vi "ManipWait.vi"(2 "Time Since Latch":u32, 3 "Instruction String":string) -> (0 "Error Out":errorcluster, 1 "Advance Trigger":bool)   [LabVIEW 2019]
uses:
  SafeParser_Integer.vi
  SafeParser_Float.vi
  SafeParser_String.vi
  dsdata.vi
  autoninfo.vi
  outputs.vi
  sensors.vi
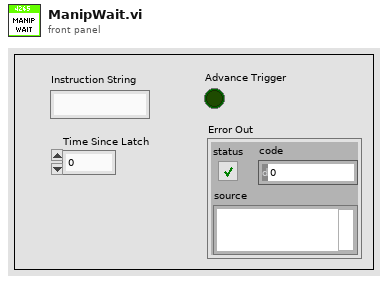
[diagram p1: front panel]
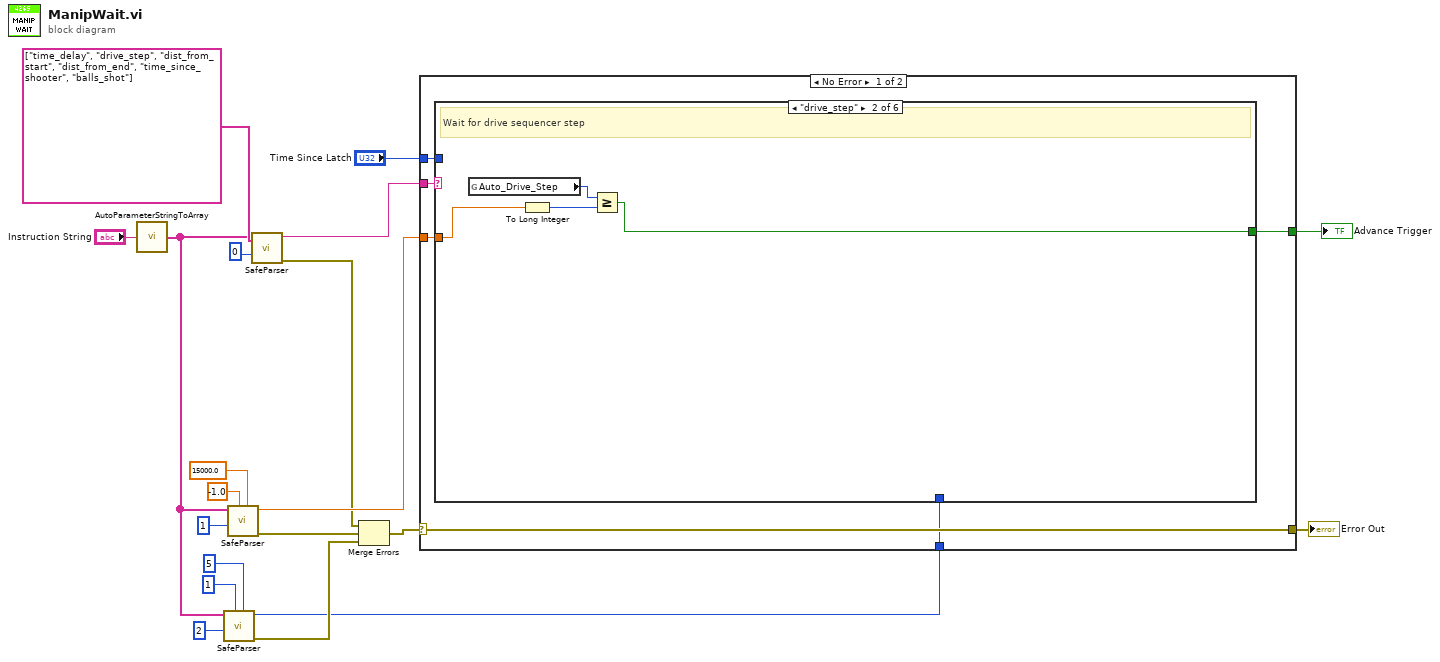
[diagram p0: block diagram]
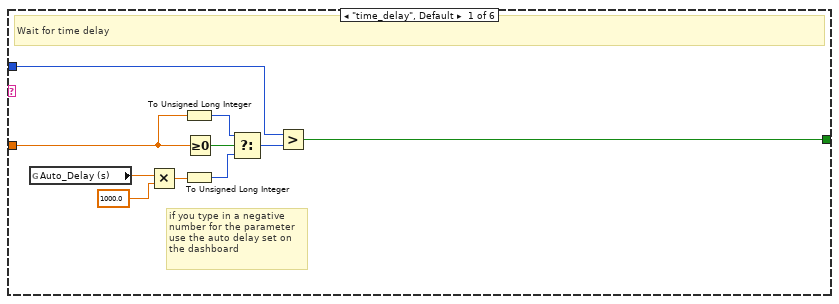
[diagram p2: hidden frame]
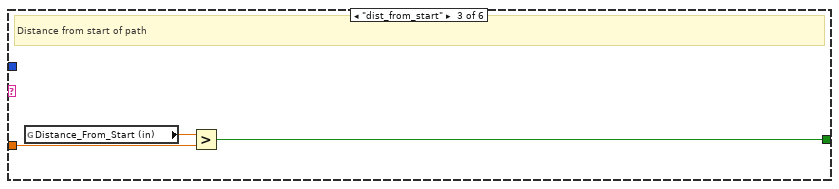
[diagram p3: hidden frame]
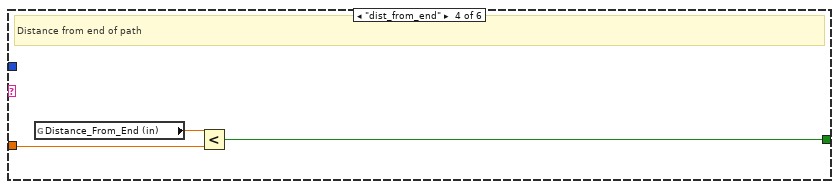
[diagram p4: hidden frame]
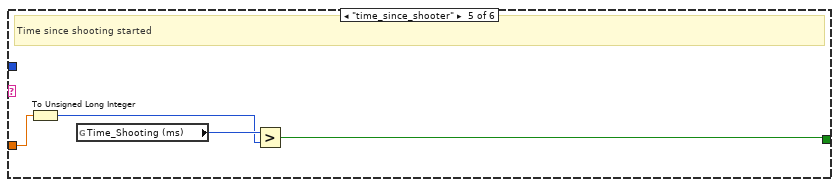
[diagram p5: hidden frame]
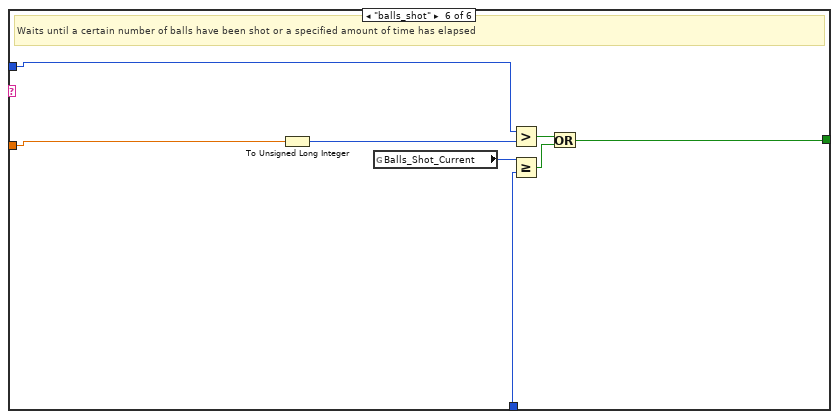
[diagram p6: hidden frame]
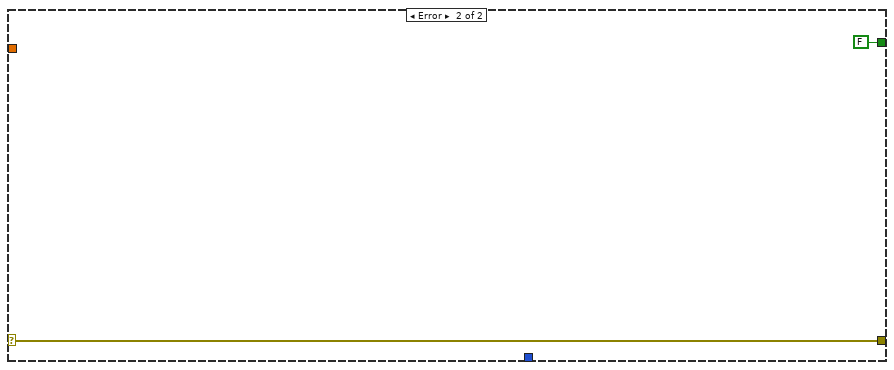
[diagram p7: hidden frame]
diagram:
  n1 = call "AutoParameterStringToArray.vi"("Parameter String"="Instruction String") -> ("Parsed Parameters"=w5:string[])
  n2 = call-poly "SafeParser.vi"("Maximum"=5, "Minimum"=1, "Array Index"=2 ("Parameter Index"), "String Array"=w5) -> ("Error Out"=w4:errorcluster, "Typecast  Value"=w3:i32)  [unwired: 6 in]
  n3 = call-poly "SafeParser.vi"("Maximum"=15000.0, "Minimum"=-1.0, "Array Index"=1 ("Parameter Index"), "String Array"=w5) -> ("Error Out"=w9:errorcluster, "Typecast  Value"=w12:dbl)  [unwired: 6 in]
  n4 = call-poly "SafeParser.vi"("Allowed Values"=string[] ["time_delay", "drive_step", "dist_from_start", "dist_from_end", "time_since_shooter", "balls_shot"], "Array Index"=0 ("Parameter Index"), "String Array"=w5) -> ("Error Out"=w8:errorcluster, "Typecast Value"=w10:string)  [unwired: 7 in]
  n5 = Merge Errors(w8, w9, w4) -> (w13:errorcluster)
  n6 = case shown="No Error" w13 {
    selector: w13 -> [w23 w59]
    tunnel: w10 -> [w26 _]
    tunnel: "Time Since Latch" -> [w25 _]
    tunnel: [w24 FALSE] -> w19
    tunnel: [w23 w59] -> w18
    tunnel: w12 -> [w22 _]
    tunnel: w3 -> [w21 _]
    frame No Error {
      n7 = case shown="\"drive_step\"" w26 {
        tunnel: w25 -> [w29 _ _ _ _ w54]
        tunnel: [w28 w38 w43 w46 w50 w53] -> w24
        tunnel: w22 -> [w27 w37 w41 w44 w47 w52]
        tunnel: w21 -> [_ _ _ _ _ w51]
        frame "time_delay", Default {
          # "if you type in a negative\nnumber for the parameter\nuse the auto delay set on \nthe dashboard"
          # "Wait for time delay"
          n8 = global read "dsdata.vi" "Auto_Delay (s)"() -> (w34:dbl)
          n9 = Multiply(x=w34, y=1000.0) -> (x*y=w35:dbl)
          n10 = To Unsigned Long Integer(number=w27) -> (unsigned 32bit integer=w33:u32)
          n11 = To Unsigned Long Integer(number=w35) -> (unsigned 32bit integer=w36:u32)
          n12 = Greater Or Equal To 0?(x=w27) -> (x >= 0?=w32:bool)
          n13 = Select(t=w33, s=w32, f=w36) -> (s? t:f=w30:u32)
          n14 = Greater?(x=w29, y=w30) -> (0:w28:bool)
        }
        frame "drive_step" {
          # "Wait for drive sequencer step"
          n15 = global read "autoninfo.vi" "Auto_Drive_Step"() -> (w40:i32)
          n16 = To Long Integer(number=w37) -> (32bit integer=w39:i32)
          n17 = Greater Or Equal?(x=w40, y=w39) -> (x >= y?=w38:bool)
        }
        frame "dist_from_start" {
          # "Distance from start of path"
          n18 = global read "autoninfo.vi" "Distance_From_Start (in)"() -> (w42:dbl)
          n19 = Greater?(x=w42, y=w41) -> (0:w43:bool)
        }
        frame "dist_from_end" {
          # "Distance from end of path"
          n20 = global read "autoninfo.vi" "Distance_From_End (in)"() -> (w45:dbl)
          n21 = Less?(x=w45, y=w44) -> (x < y?=w46:bool)
        }
        frame "time_since_shooter" {
          # "Time since shooting started"
          n22 = To Unsigned Long Integer(number=w47) -> (unsigned 32bit integer=w48:u32)
          n23 = global read "outputs.vi" "Time_Shooting (ms)"() -> (w49:u32)
          n24 = Greater?(x=w49, y=w48) -> (0:w50:bool)
        }
        frame "balls_shot" {
          # "Waits until a certain number of balls have been shot or a specified amount of time has elapsed"
          n25 = To Unsigned Long Integer(number=w52) -> (unsigned 32bit integer=w55:u32)
          n26 = global read "sensors.vi" "Balls_Shot_Current"() -> (w58:i32)
          n27 = Greater?(x=w54, y=w55) -> (0:w57:bool)
          n28 = Greater Or Equal?(x=w58, y=w51) -> (x >= y?=w56:bool)
          n29 = Or(x=w57, y=w56) -> (x .or. y?=w53:bool)
        }
      }
    }
    frame Error {
    }
  }
  "Advance Trigger" <- w19
  "Error Out" <- w18
